vi "RSSI 400 MHz Signal Strength Measurement.vi"(7 "Execute on Remote? (F)\nAKA on IMPLANT":bool, 8 "error in":errorcluster, 10 "Number of RSSI Readings":i32=1, 11 "VISA Resource Name":refnum<visa-resource-name>="COM11") -> (0 "error out":errorcluster {"code" format="%04x"}, 1 "min RSSI Value (400 MHz)":u8, 2 "mean RSSI Value (400 mHz)":dbl=nan format="%0.2f", 3 "dup VISA Resource Name":refnum<visa-resource-name>, 4 "max RSSI Value (400 MHz)":u8, 5 "400 MHz RSSI Values":u8[](array[numeric]), 6 "Timeout Reading ADC Output?":bool[](array[boolean]))   [LabVIEW 2010]
uses:
  <vilib>/Analysis/NI_AALBase.lvlib
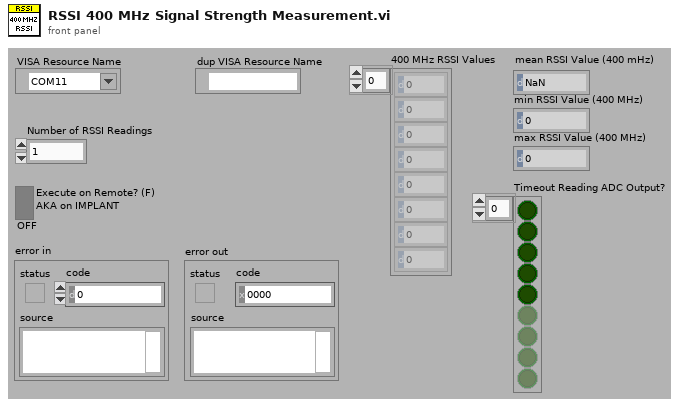
[diagram p1: front panel]
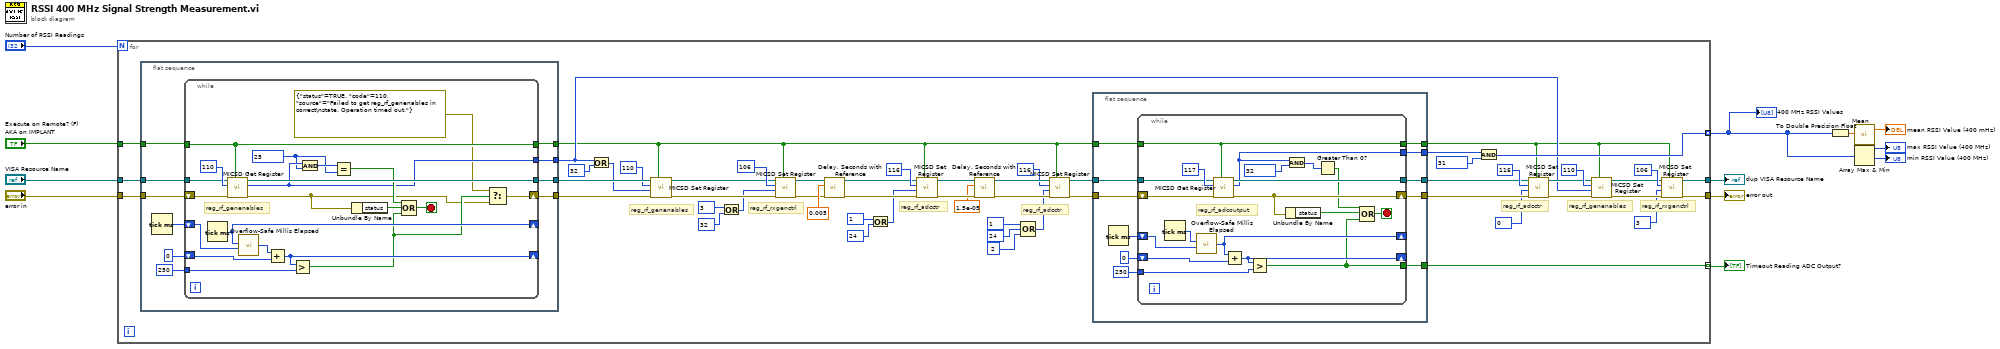
[diagram p0: block diagram]
diagram:
  n1 = for {
    N: "Number of RSSI Readings" -> [_]
    tunnel: [w19] -> w12
    tunnel: [w17] -> w11
    tunnel: [w55] -> w6 mode=indexing
    tunnel: "VISA Resource Name" -> [w54]
    tunnel: "error in" -> [w53]
    tunnel: "Execute on Remote? (F)\nAKA on IMPLANT" -> [w52]
    tunnel: [w13] -> w1 mode=indexing
    # "reg_rf_rxgenctrl"
    # "reg_rf_genenables"
    # "reg_rf_adcctr"
    # "reg_rf_adcctr"
    # "reg_rf_genenables"
    # "reg_rf_rxgenctrl"
    # "reg_rf_adcctr"
    n2 = flat-sequence {
      tunnel: w54 -> [w107]
      tunnel: w53 -> [w106]
      tunnel: w52 -> [w105]
      tunnel: [w101] -> w51
      tunnel: [w100] -> w49
      tunnel: [w99] -> w22
      tunnel: [w98] -> w15
      frame #0 {
        n3 = Tick Count (ms)() -> (millisecond timer value=w104:u32)
        n4 = while {
          tunnel: [w128] -> w101
          tunnel: w107 -> [w126]
          tunnel: w105 -> [w124]
          tunnel: [w124] -> w98
          shift-right: [w109] -> w100
          shift-left: w106 -> [w125]
          tunnel: [w120] -> w99
          tunnel: u32 250 ("y") -> [w114]
          shift-right: [w112] -> _
          shift-left: w104 -> [w116]
          shift-right: [w113] -> _
          shift-left: u32 0 ("y") -> [w115]
          stop <- w121 stop-if-true
          w118 = u8 25 ("Data")
          # "reg_rf_genenables"
          n5 = Tick Count (ms)() -> (millisecond timer value=w112:u32)
          n6 = call "MICSD Get Register.vi"("Execute on Remote?(F)"=w124, "error in (no error)"=w125, "Address"=u16 110, "VISA Resource Name"=w126) -> ("error out"=w110:errorcluster, "Data"=w120:u8, "dup VISA Resource Name"=w128:refnum<visa-resource-name>)  [unwired: 5 in]
          n7 = call "Overflow-Safe Millis Elapsed.vi"("now"=w112, "previous"=w116) -> ("elapsed"=w117:u32)  [unwired: 5 in]
          n8 = Add(x=w117, y=w115) -> (x+y=w113:u32)
          n9 = Greater?(x=w113, y=w114) -> (0:w111:bool)
          n10 = And(x=w120, y=w118) -> (x .and. y?=w119:u8)
          n11 = Equal?(x=w119, y=w118) -> (x = y?=w122:bool)
          n12 = Unbundle By Name(w110) -> ("status"=w123:bool)
          n13 = Compound Arithmetic op=OR(w122, w123, w111) -> (w121:bool)
          n14 = Select(t=errorcluster {"status"=TRUE, "code"=110, "source"="Failed to get reg_rf_genenables in correct\nstate. Operation timed out."}, s=w111, f=w110) -> (s? t:f=w109:errorcluster)
        }
      }
    }
    n15 = Or(x=w22, y=u8 32) -> (x .or. y?=w45:u8)
    n16 = call "MICSD Set Register.vi"("Execute on Remote?(F)"=w15, "error in (no error)"=w49, "Data"=w45, "Address"=u16 110, "VISA Resource Name"=w51) -> ("error out"=w48:errorcluster, "dup VISA Resource Name"=w50:refnum<visa-resource-name>)  [unwired: 5 in]
    n17 = Or(x=u8 3, y=u8 32) -> (x .or. y?=w42:u8)
    n18 = call "MICSD Set Register.vi"("Execute on Remote?(F)"=w15, "error in (no error)"=w48, "Data"=w42, "Address"=u16 106, "VISA Resource Name"=w50) -> ("error out"=w57:errorcluster, "dup VISA Resource Name"=w59:refnum<visa-resource-name>)  [unwired: 5 in]
    n19 = call "Delay, Seconds with Reference.vi"("error in"=w57, "delay"=dbl[unit] 0.005, "VISA resource"=w59) -> ("error out"=w56:errorcluster, "VISA resource dup"=w58:refnum<visa-resource-name>)  [unwired: 3 in, 1 out]
    n20 = Or(x=u8 1, y=u8 24) -> (x .or. y?=w39:u8)
    n21 = call "MICSD Set Register.vi"("Execute on Remote?(F)"=w15, "error in (no error)"=w56, "Data"=w39, "Address"=u16 116, "VISA Resource Name"=w58) -> ("error out"=w63:errorcluster, "dup VISA Resource Name"=w65:refnum<visa-resource-name>)  [unwired: 5 in]
    n22 = call "Delay, Seconds with Reference.vi"("error in"=w63, "delay"=dbl[unit] 1.5e-05, "VISA resource"=w65) -> ("error out"=w62:errorcluster, "VISA resource dup"=w64:refnum<visa-resource-name>)  [unwired: 3 in, 1 out]
    n23 = Compound Arithmetic op=OR(u8 1, u8 24, u8 2) -> (w29:u8)
    n24 = call "MICSD Set Register.vi"("Execute on Remote?(F)"=w15, "error in (no error)"=w62, "Data"=w29, "Address"=u16 116, "VISA Resource Name"=w64) -> ("error out"=w27:errorcluster, "dup VISA Resource Name"=w28:refnum<visa-resource-name>)  [unwired: 5 in]
    n25 = flat-sequence {
      tunnel: [w78] -> w36
      tunnel: [w77] -> w35
      tunnel: [w76] -> w33
      tunnel: w28 -> [w75]
      tunnel: w27 -> [w74]
      tunnel: w15 -> [w70]
      tunnel: [w69] -> w14
      tunnel: [w68] -> w13
      frame #0 {
        n26 = Tick Count (ms)() -> (millisecond timer value=w73:u32)
        n27 = while {
          tunnel: w75 -> [w96]
          tunnel: [w94] -> w78
          tunnel: w70 -> [w91]
          tunnel: [w91] -> w69
          shift-right: [w90] -> w77
          shift-left: w74 -> [w95]
          tunnel: [w89] -> w76
          tunnel: u32 250 ("y") -> [w86]
          shift-right: [w84] -> _
          shift-left: w73 -> [w87]
          shift-right: [w83] -> _
          shift-left: u32 0 ("y") -> [w85]
          tunnel: [w79] -> w68
          stop <- w80 stop-if-true
          # "reg_rf_adcoutput"
          n28 = Tick Count (ms)() -> (millisecond timer value=w88:u32)
          n29 = call "Overflow-Safe Millis Elapsed.vi"("now"=w88, "previous"=w87) -> ("elapsed"=w84:u32)  [unwired: 5 in]
          n30 = call "MICSD Get Register.vi"("Execute on Remote?(F)"=w91, "error in (no error)"=w95, "Address"=u16 117, "VISA Resource Name"=w96) -> ("error out"=w90:errorcluster, "Data"=w89:u8, "dup VISA Resource Name"=w94:refnum<visa-resource-name>)  [unwired: 5 in]
          n31 = Add(x=w84, y=w85) -> (x+y=w83:u32)
          n32 = Greater?(x=w83, y=w86) -> (0:w79:bool)
          n33 = Unbundle By Name(w90) -> ("status"=w81:bool)
          n34 = And(x=w89, y=u8 32 ("Data")) -> (x .and. y?=w92:u8)
          n35 = Greater Than 0?(x=w92) -> (x > 0?=w82:bool)
          n36 = Compound Arithmetic op=OR(w82, w81, w79) -> (w80:bool)
        }
      }
    }
    n37 = And(x=w33, y=u8 31 ("Data")) -> (x .and. y?=w55:u8)
    n38 = call "MICSD Set Register.vi"("Execute on Remote?(F)"=w14, "error in (no error)"=w35, "Data"=u8 0, "Address"=u16 116, "VISA Resource Name"=w36) -> ("error out"=w23:errorcluster, "dup VISA Resource Name"=w24:refnum<visa-resource-name>)  [unwired: 5 in]
    n39 = call "MICSD Set Register.vi"("Execute on Remote?(F)"=w14, "error in (no error)"=w23, "Data"=w22, "Address"=u16 110, "VISA Resource Name"=w24) -> ("error out"=w18:errorcluster, "dup VISA Resource Name"=w20:refnum<visa-resource-name>)  [unwired: 5 in]
    n40 = call "MICSD Set Register.vi"("Execute on Remote?(F)"=w14, "error in (no error)"=w18, "Data"=u8 3, "Address"=u16 106, "VISA Resource Name"=w20) -> ("error out"=w17:errorcluster, "dup VISA Resource Name"=w19:refnum<visa-resource-name>)  [unwired: 5 in]
  }
  "400 MHz RSSI Values" <- w6
  "dup VISA Resource Name" <- w12
  "error out" <- w11
  "Timeout Reading ADC Output?" <- w1
  n41 = To Double Precision Float(number=w6) -> (double precision float=w10:dbl[])
  n42 = call <vilib>:"Mean.vi"("X"=w10) -> ("mean"=→"mean RSSI Value (400 mHz)":dbl)  [unwired: 1 out]
  n43 = Array Max & Min(array=w6) -> (max value=→"max RSSI Value (400 MHz)":u8, min value=→"min RSSI Value (400 MHz)":u8)  [unwired: 2 out]
